vi "Begin.vi"() -> (0 "error out":errorcluster)   [LabVIEW 2012]
doc: "Called before other user functions, this VI is expected to open initial I/O refnums, load in file data, and do all program initialization. Notice that the <B>error out</B> terminal is simply used for data flow. Wiring it to other structures or subVIs ensures that this VI runs first."
uses:
  <vilib>/Rock Robotics/WPI/DriverStation/WPI_DriverStationRobotMode2.ctl
  <vilib>/Rock Robotics/WPI/Joystick/WPI_JoystickDeviceEnum.ctl
  <vilib>/Rock Robotics/WPI/Solenoid/WPI_SolenoidChannel.ctl
  <vilib>/Rock Robotics/SystemInterfaces/DIO/FPGA_DIORelayChannel.ctl
  <vilib>/Rock Robotics/WPI/Relay/WPI_RelayDirection.ctl
  <vilib>/Rock Robotics/SystemInterfaces/DIO/FPGA_DIOChannel.ctl
  <vilib>/Rock Robotics/WPI/Encoder/WPI_EncoderType.ctl
  <vilib>/Rock Robotics/SystemInterfaces/DIO/FPGA_DIOPWMChannel.ctl
  <vilib>/Rock Robotics/SystemInterfaces/AI/FPGA_AIGyroChannel.ctl
  <vilib>/Rock Robotics/SystemInterfaces/Typedef/FPGA_TypedefSolenoidModule.ctl
  Robot Global Data.vi
  <vilib>/Rock Robotics/WPI/Solenoid/WPI_SolenoidOpenSingle.vi
  <vilib>/Rock Robotics/WPI/Solenoid/Deprecated/WPI_SolenoidSetBool.vi
  <vilib>/Rock Robotics/WPI/Counter/WPI_CounterDigitalInputToDigitalSource.vi
  <vilib>/Rock Robotics/WPI/MotorControl/WPI_MotorControlOpen Jaguar.vi
  <vilib>/Rock Robotics/WPI/RobotDrive/WPI_RobotDriveOpen4MotorWithTalon.vi
  <vilib>/Rock Robotics/WPI/Compressor/WPI_CompressorGetSetRefNum.vi
  <vilib>/Rock Robotics/WPI/MotorControl/WPI_MotorControlOpen Talon.vi
  <vilib>/Rock Robotics/WPI/RobotDrive/WPI_RobotDriveOpen4MotorWithExistingMotors.vi
  <vilib>/Rock Robotics/WPI/MotorControl/WPI_MotorControlOpen Victor.vi
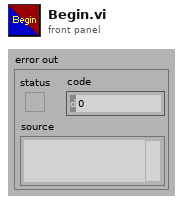
[diagram p1: front panel]
types:
  T1 = typedef "FPGA_DIOChannel.ctl" = enum8{"DIO 1", "DIO 2", "DIO 3", "DIO 4", "DIO 5", "DIO 6", "DIO 7", "DIO 8", "DIO 9", "DIO 10", "DIO 11", "DIO 12", "DIO 13", "DIO 14", "Invalid"}
  T2 = typedef "WPI_SolenoidChannel.ctl" = enum8{"Solenoid 1", "Solenoid 2", "Solenoid 3", "Solenoid 4", "Solenoid 5", "Solenoid 6", "Solenoid 7", "Solenoid 8", "Invalid"}
  T3 = typedef "FPGA_TypedefSolenoidModule.ctl" = enum16{"Solenoid Module 1", "Solenoid Module 2"}
  T4 = typedef "FPGA_AIGyroChannel.ctl" = enum8{"AI 1", "AI 2", "Invalid"}
  T5 = typedef "WPI_EncoderType.ctl" = enum16{"1x", "2x", "4x"}
  T6 = typedef "FPGA_DIORelayChannel.ctl" = enum8{"Relay 1", "Relay 2", "Relay 3", "Relay 4", "Relay 5", "Relay 6", "Relay 7", "Relay 8", "Invalid"}
  T7 = typedef "WPI_JoystickDeviceEnum.ctl" = enum16{"USB 1", "USB 2", "USB 3", "USB 4", "Kinect 1", "Kinect 2"}
  T8 = typedef "FPGA_DIOPWMChannel.ctl" = enum8{"PWM 1", "PWM 2", "PWM 3", "PWM 4", "PWM 5", "PWM 6", "PWM 7", "PWM 8", "PWM 9", "PWM 10", "Invalid"}
  T9 = typedef "WPI_RelayDirection.ctl" = enum16{"Both directions", "Forward only", "Reverse only"}
  T10 = typedef "WPI_DriverStationRobotMode2.ctl" = enum16{"Autonomous Disabled", "Autonomous Enabled", "Teleop Disabled", "Teleop Enabled", "Timeout", "Finish", "Test Disabled", "Test Enabled"}
  T11 = typedef "WPI_RobotDriveDevRef.ctl" = cluster{"DevStatus":errorcluster, "Motors[]":T12[], "Square Inputs":bool, "Max Output":dbl, "Isochronous":bool}
  T12 = typedef "WPI_MotorControlDeviceRef.ctl" = cluster{"DeviceStatus":errorcluster, "Type":enum16{"PWM", "CAN"}, "PWM":cluster{"Digital Module":T13, "PWM Channel":T8, "DeadBand":T14}, "CAN":cluster{"Device Number":u8, "Control Mode":T15, "Semaphore":T16, "Max Vout":dbl}, "Invert":bool, "TransformRef":T17, "InvTransformRef":T17}
  T13 = typedef "FPGA_TypedefDigitalModule.ctl" = enum16{"Digital Module 1", "Digital Module 2"}
  T14 = typedef "WPI_PWMDeadband.ctl" = cluster{"Name":string, "maxPositivePwm":i32, "minPositivePwm":i32, "centerPwm":i32, "maxNegativePwm":i32, "minNegativePwm":i32, "angularRange":u16}
  T15 = typedef "WPI_CANJaguar_ControlMode.ctl" = enum8{"Percent VBus", "Current", "Speed", "Position", "Voltage"}
  T16 = typedef "Semaphore RefNum" = refnum<k1>
  T17 = typedef "WPI_PWMTransform_ConPane.ctl" = refnum<vi>
  T18 = typedef "WPI_DigitalInputDevRef.ctl" = cluster{"DevStatus":errorcluster, "DIO Channel":T1, "Digital Module":T13}
  T19 = typedef "WPI_CompressorDevRef.ctl" = cluster{"DevStatus":errorcluster, "DigitalInputDevRef":T18, "RelayDevRef":T20}
  T20 = typedef "WPI_RelayDevRef.ctl" = cluster{"DevStatus":errorcluster, "Relay Channel":T6, "Digital Module":T13, "Relay Direction":T9}
  T21 = typedef "WPI_JoystickDevRef.ctl" = cluster{"Device":T7}
  T22 = typedef "WPI_SolenoidDevRef.ctl" = cluster{"DevStatus":errorcluster, "Solenoid Module":T3, "Forward Solenoid Channel":T2, "Reverse Solenoid Channel":T2}
  T23 = typedef "FPGA_CounterEncoderSourceConvertionLVSourceType.ctl" = cluster{"DevStatus":errorcluster, "AnalogTriggerMode?":bool, "DigitalMode":cluster{"Digital Module":T13, "DIO Channel":T24}, "AnalogTriggerMode":cluster{"AnalogTriggerIndex":T25, "OutputType":T26}}
  T24 = typedef "FPGA_DIODigitalSourceChannel.ctl" = enum8{"DIO 1", "DIO 2", "DIO 3", "DIO 4", "DIO 5", "DIO 6", "DIO 7", "DIO 8", "DIO 9", "DIO 10", "DIO 11", "DIO 12", "DIO 13", "DIO 14", "Disabled"}
  T25 = typedef "FPGA_AnalogTriggerIndex.ctl" = enum8{"Trig 0", "Trig 1", "Trig 2", "Trig 3", "Trig 4", "Trig 5", "Trig 6", "Trig 7", "Invalid"}
  T26 = typedef "FPGA_AnalogTriggerOutType.ctl" = enum16{"InWindow", "TriggerState", "Rising", "Falling"}
  T27 = typedef "WPI_GyroDevRef.ctl" = cluster{"DevStatus":errorcluster, "Analog Module":T28, "Analog Channel":T29, "Offset":dbl, "Gain (VoltsPerDegree/Second)":dbl}
  T28 = typedef "FPGA_TypedefAnalogModule.ctl" = enum16{"Analog Module 1", "Analog Module 2"}
  T29 = typedef "FPGA_AIChannel.ctl" = enum8{"AI 1", "AI 2", "AI 3", "AI 4", "AI 5", "AI 6", "AI 7", "AI 8", "Invalid"}
  T30 = typedef "WPI_EncoderDevRef.ctl" = cluster{"DevStatus":errorcluster, "EncoderIndex":T31, "CounterIndex":T32, "DistancePerCount":dbl, "Decoding Type":T5}
  T31 = typedef "FPGA_EncoderIdx.ctl" = enum8{"Enc 0", "Enc 1", "Enc 2", "Enc 3", "Invalid"}
  T32 = typedef "FPGA_CounterCtrSystemIndex.ctl" = enum8{"Ctr 0", "Ctr 1", "Ctr 2", "Ctr 3", "Ctr 4", "Ctr 5", "Ctr 6", "Ctr 7", "Invalid"}
  T33 = cluster{"Target Voltage":dbl, "Target Speed":dbl, "Angle Up?":bool}
  T34 = cluster{"Target Voltage":dbl, "Target Speed":i32, "Angle Up?":bool}
  T35 = cluster{"Target Voltage":i32, "Target Speed":i32, "Angle Up?":bool}
  T36 = cluster{"Target Voltage":dbl, "Target Speed":dbl, "Angle Up?":bool}[]
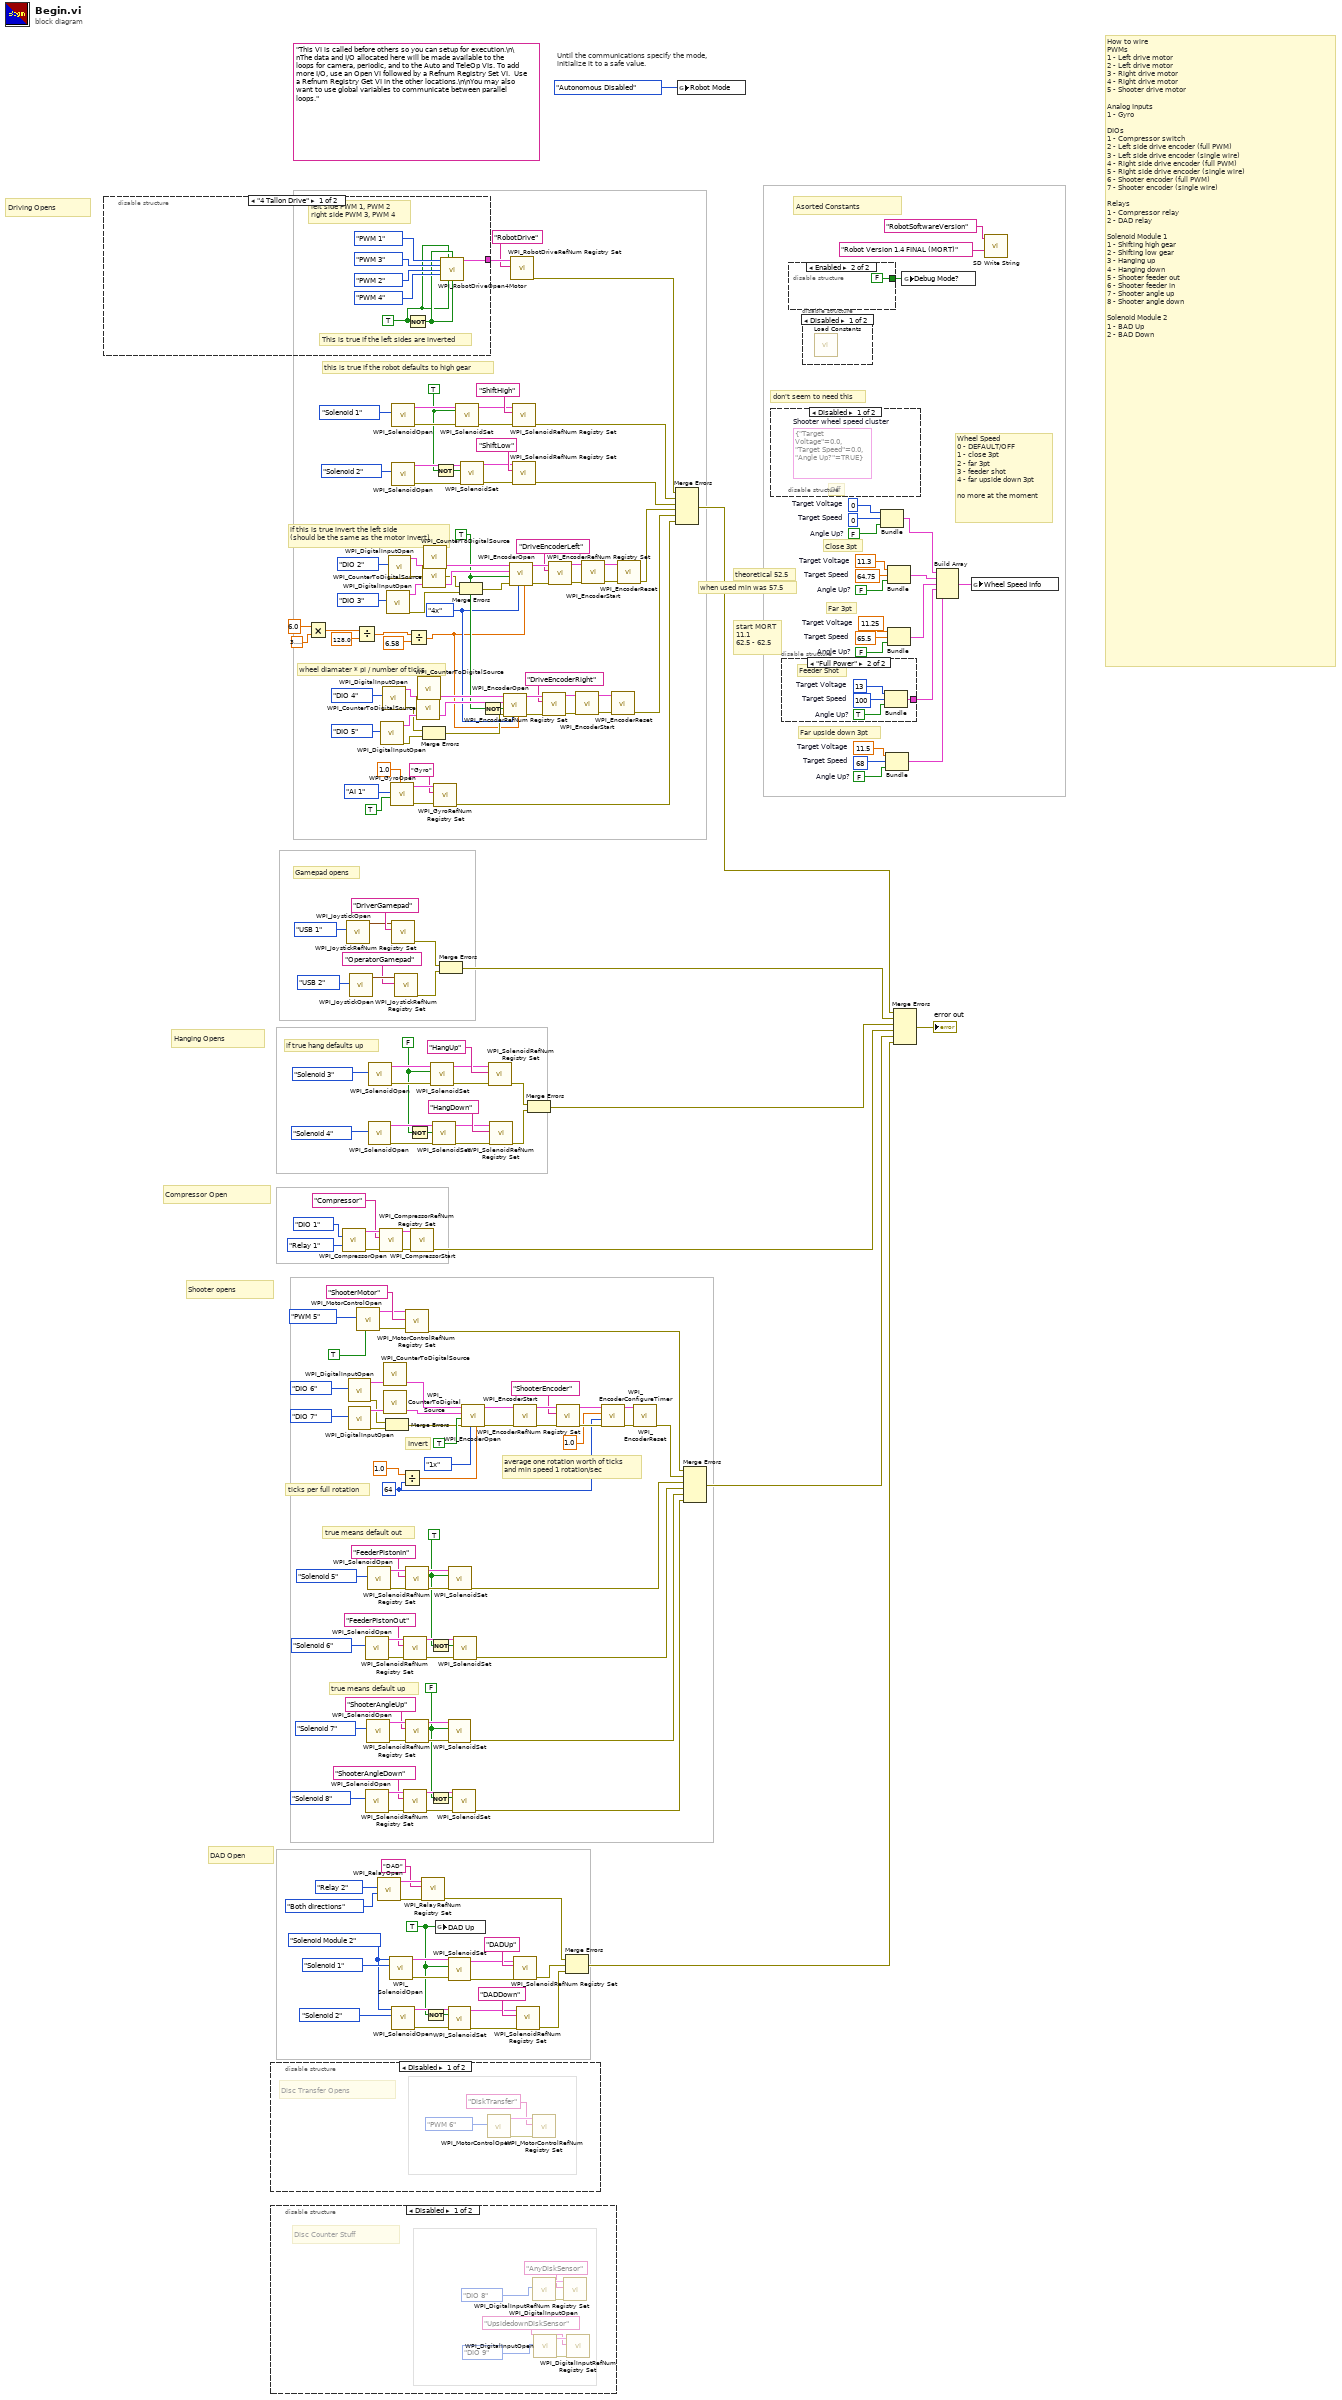
[diagram p0: block diagram]
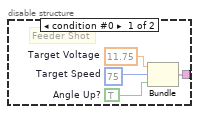
[diagram p3: hidden frame]
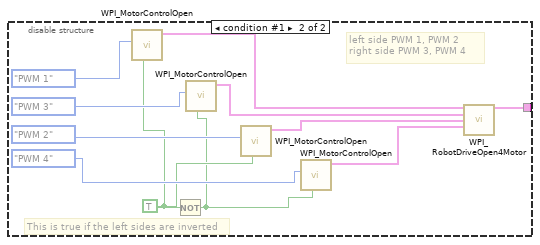
[diagram p4: hidden frame]
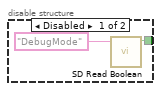
[diagram p5: hidden frame]
diagram:
  w6 = FALSE  # Angle Up?
  w5 = 65.5  # Target Speed
  w4 = 11.25  # Target Voltage
  w10 = FALSE  # Angle Up?
  w9 = 68  # Target Speed
  w8 = 11.5  # Target Voltage
  w14 = FALSE  # Angle Up?
  w13 = 0  # Target Speed
  w12 = 0  # Target Voltage
  w16 = u8 64 ("Number Samples to Average")
  w23 = FALSE  # Angle Up?
  w24 = 64.75  # Target Speed
  w25 = 11.3  # Target Voltage
  w84 = FALSE
  w98 = TRUE
  w60 = TRUE
  w62 = FPGA_TypedefSolenoidModule."Solenoid Module 2" ("Solenoid Module (Module 1)")
  w63 = FALSE
  w65 = WPI_EncoderType."4x" ("Decoding Type")
  w66 = TRUE ("Invert Direction (False)")
  w82 = TRUE
  (unwired) "This VI is called before others so you can setup for execution.\n\nThe data and I/O allocated here will be made available to the loops for camera, periodic, and to the Auto and TeleOp VIs. To add more I/O, use an Open VI followed by a Refnum Registry Set VI.  Use a Refnum Registry Get VI in the other locations.\n\nYou may also want to use global variables to communicate between parallel loops."
  # "start MORT\n11.1\n62.5 - 62.5"
  # "when used min was 57.5"
  # "theoretical 52.5"
  # "don't seem to need this"
  # "Far 3pt"
  # "Far upside down 3pt"
  # "average one rotation worth of ticks\nand min speed 1 rotation/sec"
  # "Close 3pt"
  # "How to wire\nPWMs\n1 - Left drive motor\n2 - Left drive motor\n3 - Right drive motor\n4 - Right drive motor\n5 - Shooter drive motor\n\nAnalog Inputs\n1 - Gyro\n\nDIOs\n1 - Compressor switch\n2 - Left side drive encoder (full PWM)\n3 - Left side drive encoder (single wire)\n4 - Right side drive encoder (full PWM)\n5 - Right side drive encoder (single wire)\n6 - Shooter encoder (full PWM)\n7 - Shooter encoder (single wire)\n\nRelays\n1 - Compressor relay\n2 - DAD relay\n\nSolenoid Module 1\n1 - Shifting high gear\n2 - Shifting low gear\n3 - Hanging up\n4 - Hanging down\n5 - Shooter feeder out\n6 - Shooter feeder in\n7 - Shooter angle up\n8 - Shooter angle down\n\nSolenoid Module 2\n1 - BAD Up\n2 - BAD Down"
  # "Asorted Constants"
  # "true means default up"
  # "true means default out"
  # "if true hang defaults up"
  # "Gamepad opens"
  # "wheel diamater * pi / number of ticks"
  # "if this is true invert the left side\n(should be the same as the motor invert)"
  # "this is true if the robot defaults to high gear"
  # "Compressor Open"
  # "Wheel Speed\n0 - DEFAULT/OFF\n1 - close 3pt\n2 - far 3pt\n3 - feeder shot\n4 - far upside down 3pt\n\nno more at the moment"
  # "DAD Open"
  # "Hanging Opens"
  # "Driving Opens"
  # "Shooter opens"
  # "Invert"
  # "ticks per full rotation"
  # "Until the communications specify the mode,\ninitialize it to a safe value."
  n1 = disable-structure shown="\"4 Tallon Drive\"" {
    disable-tunnel: [w219 w234] -> w212
    frame condition #0 (active) {
      w217 = TRUE ("Rear Left Motor Inverted")
      # "left side PWM 1, PWM 2\nright side PWM 3, PWM 4"
      # "This is true if the left sides are inverted"
      n2 = Not(x=w217) -> (.not. x?=w218:bool)
      n3 = call-poly <vilib>:"WPI_RobotDriveOpen4Motor.vi"("Rear Left Motor"=FPGA_DIOPWMChannel."PWM 1", "Rear Left Motor Inverted"=w217, "Rear Right Motor Inverted"=w218, "Rear Right Motor"=FPGA_DIOPWMChannel."PWM 3", "Front Left Motor"=FPGA_DIOPWMChannel."PWM 2", "Front Right Motor"=FPGA_DIOPWMChannel."PWM 4" ("Front Left Motor"), "Front Left Motor Inverted"=w217, "Front Right Motor Inverted"=w218) -> ("RobotDriveDevRef"=w219:T11)  [unwired: 6 in, 1 out]
    }
    frame condition #1 {
      w229 = TRUE ("Rear Left Motor Inverted")
      # "left side PWM 1, PWM 2\nright side PWM 3, PWM 4"
      # "This is true if the left sides are inverted"
      n4 = call-poly <vilib>:"WPI_MotorControlOpen.vi"("Invert"=w229, "PWM Channel"=FPGA_DIOPWMChannel."PWM 1" ("Rear Left Motor")) -> ("MotorControlDeviceRef"=w227:T12)  [unwired: 8 in, 1 out]
      n5 = Not(x=w229) -> (.not. x?=w228:bool)
      n6 = call-poly <vilib>:"WPI_MotorControlOpen.vi"("Invert"=w228, "PWM Channel"=FPGA_DIOPWMChannel."PWM 3" ("Rear Right Motor")) -> ("MotorControlDeviceRef"=w226:T12)  [unwired: 8 in, 1 out]
      n7 = call-poly <vilib>:"WPI_MotorControlOpen.vi"("Invert"=w229, "PWM Channel"=FPGA_DIOPWMChannel."PWM 2" ("Front Left Motor")) -> ("MotorControlDeviceRef"=w225:T12)  [unwired: 8 in, 1 out]
      n8 = call-poly <vilib>:"WPI_MotorControlOpen.vi"("Invert"=w228, "PWM Channel"=FPGA_DIOPWMChannel."PWM 4" ("Front Left Motor")) -> ("MotorControlDeviceRef"=w224:T12)  [unwired: 8 in, 1 out]
      n9 = call-poly <vilib>:"WPI_RobotDriveOpen4Motor.vi"("Rear Left Motor Dev Ref"=w227, "Rear Right Motor Dev Ref"=w226, "Front Left Motor Dev Ref"=w225, "Front Right Motor Dev Ref"=w224) -> ("RobotDriveDevRef"=w234:T11)  [unwired: 10 in, 1 out]
    }
  }
  n10 = disable-structure shown="Disabled" {
    frame Disabled {
      # "Disc Transfer Opens"
      n11 = call-poly <vilib>:"WPI_MotorControlOpen.vi"("PWM Channel"=FPGA_DIOPWMChannel."PWM 6") -> ("error out"=w236:errorcluster, "MotorControlDeviceRef"=w237:T12)  [unwired: 9 in]
      n12 = call <vilib>:"WPI_MotorControlRefNum Registry Set.vi"("error in (no error)"=w236, "refnum name"="DiskTransfer", "MotorControlDevRef"=w237) -> ()  [unwired: 7 in, 2 out]
    }
    frame Enabled {
    }
  }
  n13 = disable-structure shown="Disabled" {
    frame Disabled {
      # "Disc Counter Stuff"
      n14 = call <vilib>:"WPI_DigitalInputOpen.vi"("DIO Channel"=FPGA_DIOChannel."DIO 8") -> ("error out"=w246:errorcluster, "DigitalInputDevRef"=w245:T18)  [unwired: 9 in]
      n15 = call <vilib>:"WPI_DigitalInputOpen.vi"("DIO Channel"=FPGA_DIOChannel."DIO 9") -> ("error out"=w244:errorcluster, "DigitalInputDevRef"=w243:T18)  [unwired: 9 in]
      n16 = call <vilib>:"WPI_DigitalInputRefNum Registry Set.vi"("error in (no error)"=w246, "refnum name"="AnyDiskSensor", "DigitalInputDevRef"=w245) -> ()  [unwired: 7 in, 2 out]
      n17 = call <vilib>:"WPI_DigitalInputRefNum Registry Set.vi"("error in (no error)"=w244, "refnum name"="UpsidedownDiskSensor", "DigitalInputDevRef"=w243) -> ()  [unwired: 7 in, 2 out]
    }
    frame Enabled {
    }
  }
  n18 = Multiply(x=6.0, y=3.141592653589793) -> (x*y=w151:dbl)
  n19 = call <vilib>:"WPI_CompressorOpen.vi"("Pressure Switch DIO Channel"=FPGA_DIOChannel."DIO 1", "Relay Channel"=FPGA_DIORelayChannel."Relay 1") -> ("CompressorDevRef"=w164:T19, "error out"=w162:errorcluster)  [unwired: 12 in]
  n20 = call <vilib>:"WPI_JoystickOpen.vi"("JoystickDevice"=WPI_JoystickDeviceEnum."USB 1") -> ("JoystickDevRef"=w214:T21)  [unwired: 10 in]
  n21 = call <vilib>:"WPI_DigitalInputOpen.vi"("DIO Channel"=FPGA_DIOChannel."DIO 6") -> ("error out"=w180:errorcluster, "DigitalInputDevRef"=w193:T18)  [unwired: 9 in]
  n22 = call <vilib>:"WPI_DigitalInputOpen.vi"("DIO Channel"=FPGA_DIOChannel."DIO 7") -> ("error out"=w179:errorcluster, "DigitalInputDevRef"=w189:T18)  [unwired: 9 in]
  n23 = call <vilib>:"WPI_JoystickOpen.vi"("JoystickDevice"=WPI_JoystickDeviceEnum."USB 2") -> ("JoystickDevRef"=w166:T21)  [unwired: 10 in]
  n24 = Divide(x=w151, y=128.0 ("x")) -> (x/y=w2:dbl)
  n25 = call-poly <vilib>:"WPI_MotorControlOpen.vi"("Invert"=TRUE, "PWM Channel"=FPGA_DIOPWMChannel."PWM 5") -> ("error out"=w173:errorcluster, "MotorControlDeviceRef"=w174:T12)  [unwired: 8 in]
  n26 = call-poly <vilib>:"WPI_SolenoidOpen.vi"("Solenoid Channel"=WPI_SolenoidChannel."Solenoid 8") -> ("error out"=w94:errorcluster, "SolenoidDevRef"=w93:T22)  [unwired: 9 in]
  n27 = call-poly <vilib>:"WPI_SolenoidOpen.vi"("Solenoid Channel"=WPI_SolenoidChannel."Solenoid 6") -> ("error out"=w108:errorcluster, "SolenoidDevRef"=w107:T22)  [unwired: 9 in]
  n28 = call-poly <vilib>:"WPI_SolenoidOpen.vi"("Solenoid Channel"=WPI_SolenoidChannel."Solenoid 7") -> ("error out"=w89:errorcluster, "SolenoidDevRef"=w90:T22)  [unwired: 9 in]
  n29 = call-poly <vilib>:"WPI_SolenoidOpen.vi"("Solenoid Channel"=WPI_SolenoidChannel."Solenoid 5") -> ("error out"=w103:errorcluster, "SolenoidDevRef"=w104:T22)  [unwired: 9 in]
  n30 = call-poly <vilib>:"WPI_SolenoidOpen.vi"("Solenoid Channel"=WPI_SolenoidChannel."Solenoid 4") -> ("error out"=w130:errorcluster, "SolenoidDevRef"=w131:T22)  [unwired: 9 in]
  n31 = call-poly <vilib>:"WPI_SolenoidOpen.vi"("Solenoid Channel"=WPI_SolenoidChannel."Solenoid 3") -> ("error out"=w133:errorcluster, "SolenoidDevRef"=w132:T22)  [unwired: 9 in]
  n32 = call <vilib>:"WPI_RelayOpen.vi"("Relay Direction"=WPI_RelayDirection."Both directions", "Relay Channel"=FPGA_DIORelayChannel."Relay 2") -> ("error out"=w196:errorcluster, "RelayDevRef"=w195:T20)  [unwired: 8 in]
  n33 = call <vilib>:"WPI_CompressorRefNum Registry Set.vi"("error in (no error)"=w162, "refnum name"="Compressor", "CompressorDevRef"=w164) -> ("error out"=w112:errorcluster, "CompressorDevRef"=w113:T19)  [unwired: 7 in]
  n34 = call <vilib>:"WPI_DigitalInputOpen.vi"("DIO Channel"=FPGA_DIOChannel."DIO 5") -> ("error out"=w53:errorcluster, "DigitalInputDevRef"=w74:T18)  [unwired: 9 in]
  n35 = call <vilib>:"WPI_DigitalInputOpen.vi"("DIO Channel"=FPGA_DIOChannel."DIO 4") -> ("error out"=w52:errorcluster, "DigitalInputDevRef"=w73:T18)  [unwired: 9 in]
  n36 = call-poly <vilib>:"WPI_CounterToDigitalSource.vi"("DigitalInputDevRef"=w193) -> ("Digital Source"=w192:T23)  [unwired: 6 in]
  n37 = call-poly <vilib>:"WPI_CounterToDigitalSource.vi"("DigitalInputDevRef"=w189) -> ("Digital Source"=w186:T23)  [unwired: 6 in]
  n38 = Merge Errors(w180, w179) -> (w181:errorcluster)
  n39 = call <vilib>:"WPI_DigitalInputOpen.vi"("DIO Channel"=FPGA_DIOChannel."DIO 3") -> ("error out"=w48:errorcluster, "DigitalInputDevRef"=w154:T18)  [unwired: 9 in]
  n40 = call <vilib>:"WPI_DigitalInputOpen.vi"("DIO Channel"=FPGA_DIOChannel."DIO 2") -> ("error out"=w49:errorcluster, "DigitalInputDevRef"=w155:T18)  [unwired: 9 in]
  n41 = call-poly <vilib>:"WPI_SolenoidOpen.vi"("Solenoid Channel"=WPI_SolenoidChannel."Solenoid 1", "Solenoid Module (Module 1)"=w62) -> ("error out"=w117:errorcluster, "SolenoidDevRef"=w121:T22)  [unwired: 8 in]
  n42 = call <vilib>:"WPI_GyroOpen.vi"("Calibration Time (s)"=1.0, "Calibrate On Open"=TRUE, "Analog Channel"=FPGA_AIGyroChannel."AI 1") -> ("error out"=w143:errorcluster, "GyroDevRef"=w142:T27)  [unwired: 6 in, 1 out]
  n43 = call-poly <vilib>:"WPI_SolenoidOpen.vi"("Solenoid Channel"=WPI_SolenoidChannel."Solenoid 1") -> ("error out"=w203:errorcluster, "SolenoidDevRef"=w206:T22)  [unwired: 9 in]
  n44 = call-poly <vilib>:"WPI_SolenoidOpen.vi"("Solenoid Channel"=WPI_SolenoidChannel."Solenoid 2") -> ("error out"=w200:errorcluster, "SolenoidDevRef"=w202:T22)  [unwired: 9 in]
  n45 = call <vilib>:"WPI_JoystickRefNum Registry Set.vi"("refnum name"="DriverGamepad", "JoystickDevRef"=w214) -> ("error out"=w45:errorcluster)  [unwired: 8 in, 1 out]
  n46 = call-poly <vilib>:"WPI_SolenoidOpen.vi"("Solenoid Channel"=WPI_SolenoidChannel."Solenoid 2", "Solenoid Module (Module 1)"=w62) -> ("error out"=w114:errorcluster, "SolenoidDevRef"=w119:T22)  [unwired: 8 in]
  n47 = call <vilib>:"WPI_JoystickRefNum Registry Set.vi"("refnum name"="OperatorGamepad", "JoystickDevRef"=w166) -> ("error out"=w44:errorcluster)  [unwired: 8 in, 1 out]
  n48 = Divide(x=1.0, y=w16) -> (x/y=w17:dbl)
  n49 = call <vilib>:"WPI_SolenoidRefNum Registry Set.vi"("error in (no error)"=w108, "refnum name"="FeederPistonOut", "SolenoidDevRef"=w107) -> ("error out"=w110:errorcluster, "SolenoidDevRef"=w109:T22)  [unwired: 7 in]
  n50 = call <vilib>:"WPI_SolenoidRefNum Registry Set.vi"("error in (no error)"=w94, "refnum name"="ShooterAngleDown", "SolenoidDevRef"=w93) -> ("error out"=w96:errorcluster, "SolenoidDevRef"=w95:T22)  [unwired: 7 in]
  n51 = call <vilib>:"WPI_MotorControlRefNum Registry Set.vi"("error in (no error)"=w173, "refnum name"="ShooterMotor", "MotorControlDevRef"=w174) -> ("error out"=w41:errorcluster)  [unwired: 7 in, 1 out]
  n52 = call <vilib>:"WPI_SolenoidRefNum Registry Set.vi"("error in (no error)"=w103, "refnum name"="FeederPistonIn", "SolenoidDevRef"=w104) -> ("error out"=w101:errorcluster, "SolenoidDevRef"=w102:T22)  [unwired: 7 in]
  n53 = call <vilib>:"WPI_SolenoidRefNum Registry Set.vi"("error in (no error)"=w89, "refnum name"="ShooterAngleUp", "SolenoidDevRef"=w90) -> ("error out"=w87:errorcluster, "SolenoidDevRef"=w88:T22)  [unwired: 7 in]
  n54 = Divide(x=w2, y=6.58 ("x")) -> (x/y=w3:dbl)
  n55 = Not(x=w63) -> (.not. x?=w64:bool)
  n56 = call <vilib>:"WPI_CompressorStart.vi"("error in (no error)"=w112, "CompressorDevRef"=w113) -> ("error out"=w29:errorcluster)  [unwired: 8 in, 1 out]
  n57 = call-poly <vilib>:"WPI_CounterToDigitalSource.vi"("DigitalInputDevRef"=w74) -> ("Digital Source"=w71:T23)  [unwired: 6 in]
  n58 = call-poly <vilib>:"WPI_CounterToDigitalSource.vi"("DigitalInputDevRef"=w73) -> ("Digital Source"=w69:T23)  [unwired: 6 in]
  n59 = call <vilib>:"WPI_RelayRefNum Registry Set.vi"("error in (no error)"=w196, "refnum name"="DAD", "RelayDevRef"=w195) -> ("error out"=w35:errorcluster)  [unwired: 7 in, 1 out]
  n60 = Merge Errors(w52, w53) -> (w51:errorcluster)
  n61 = call-poly <vilib>:"WPI_CounterToDigitalSource.vi"("DigitalInputDevRef"=w154) -> ("Digital Source"=w157:T23)  [unwired: 6 in]
  n62 = call-poly <vilib>:"WPI_CounterToDigitalSource.vi"("DigitalInputDevRef"=w155) -> ("Digital Source"=w159:T23)  [unwired: 6 in]
  n63 = Not(x=w60) -> (.not. x?=w61:bool)
  n64 = Not(x=w84) -> (.not. x?=w97:bool)
  n65 = Not(x=w98) -> (.not. x?=w111:bool)
  n66 = call-poly <vilib>:"WPI_SolenoidSet.vi"("error in (no error)"=w133, "Value"=w63, "SolenoidDevRef"=w132) -> ("error out"=w126:errorcluster, "SolenoidDevRef"=w129:T22)  [unwired: 7 in]
  n67 = call-poly <vilib>:"WPI_SolenoidSet.vi"("error in (no error)"=w130, "Value"=w64, "SolenoidDevRef"=w131) -> ("error out"=w127:errorcluster, "SolenoidDevRef"=w128:T22)  [unwired: 7 in]
  n68 = Not(x=w82) -> (.not. x?=w83:bool)
  n69 = call <vilib>:"WPI_GyroRefNum Registry Set.vi"("error in (no error)"=w143, "refnum name"="Gyro", "GyroDevRef"=w142) -> ("error out"=w46:errorcluster)  [unwired: 7 in, 1 out]
  n70 = global write "Robot Global Data.vi" "DAD Up"(w60) -> ()
  n71 = Merge Errors(w45, w44) -> (w31:errorcluster)
  n72 = call-poly <vilib>:"WPI_SolenoidSet.vi"("error in (no error)"=w87, "Value"=w84, "SolenoidDevRef"=w88) -> ("error out"=w37:errorcluster)  [unwired: 7 in, 1 out]
  n73 = call-poly <vilib>:"WPI_SolenoidSet.vi"("error in (no error)"=w117, "Value"=w60, "SolenoidDevRef"=w121) -> ("error out"=w116:errorcluster, "SolenoidDevRef"=w120:T22)  [unwired: 7 in]
  n74 = call-poly <vilib>:"WPI_SolenoidSet.vi"("error in (no error)"=w114, "Value"=w61, "SolenoidDevRef"=w119) -> ("error out"=w115:errorcluster, "SolenoidDevRef"=w118:T22)  [unwired: 7 in]
  n75 = call-poly <vilib>:"WPI_SolenoidSet.vi"("error in (no error)"=w101, "Value"=w98, "SolenoidDevRef"=w102) -> ("error out"=w39:errorcluster)  [unwired: 7 in, 1 out]
  n76 = call-poly <vilib>:"WPI_SolenoidSet.vi"("error in (no error)"=w96, "Value"=w97, "SolenoidDevRef"=w95) -> ("error out"=w36:errorcluster)  [unwired: 7 in, 1 out]
  n77 = call-poly <vilib>:"WPI_SolenoidSet.vi"("error in (no error)"=w110, "Value"=w111, "SolenoidDevRef"=w109) -> ("error out"=w38:errorcluster)  [unwired: 7 in, 1 out]
  n78 = call-poly <vilib>:"WPI_SolenoidSet.vi"("error in (no error)"=w203, "Value"=w82, "SolenoidDevRef"=w206) -> ("error out"=w204:errorcluster, "SolenoidDevRef"=w205:T22)  [unwired: 7 in]
  n79 = Merge Errors(w49, w48) -> (w50:errorcluster)
  n80 = call-poly <vilib>:"WPI_SolenoidSet.vi"("error in (no error)"=w200, "Value"=w83, "SolenoidDevRef"=w202) -> ("error out"=w199:errorcluster, "SolenoidDevRef"=w201:T22)  [unwired: 7 in]
  n81 = call <vilib>:"WPI_EncoderOpen.vi"("DistancePerCount"=w17, "Decoding Type"=WPI_EncoderType."1x", "error in (no error)"=w181, "Invert Direction (False)"=TRUE, "BSource"=w186, "ASource"=w192) -> ("error out"=w182:errorcluster, "EncoderDevRef"=w183:T30)  [unwired: 4 in]
  n82 = Not(x=w66) -> (.not. x?=w67:bool)
  n83 = call <vilib>:"WPI_SolenoidRefNum Registry Set.vi"("error in (no error)"=w126, "refnum name"="HangUp", "SolenoidDevRef"=w129) -> ("error out"=w43:errorcluster)  [unwired: 7 in, 1 out]
  n84 = call <vilib>:"WPI_SolenoidRefNum Registry Set.vi"("error in (no error)"=w127, "refnum name"="HangDown", "SolenoidDevRef"=w128) -> ("error out"=w42:errorcluster)  [unwired: 7 in, 1 out]
  n85 = call <vilib>:"WPI_EncoderOpen.vi"("DistancePerCount"=w3, "Decoding Type"=w65, "error in (no error)"=w51, "Invert Direction (False)"=w67, "BSource"=w71, "ASource"=w69) -> ("error out"=w75:errorcluster, "EncoderDevRef"=w76:T30)  [unwired: 4 in]
  n86 = call <vilib>:"WPI_EncoderOpen.vi"("DistancePerCount"=w3, "Decoding Type"=w65, "error in (no error)"=w50, "Invert Direction (False)"=w66, "BSource"=w157, "ASource"=w159) -> ("error out"=w150:errorcluster, "EncoderDevRef"=w149:T30)  [unwired: 4 in]
  n87 = call <vilib>:"WPI_RobotDriveRefNum Registry Set.vi"("refnum name"="RobotDrive", "RobotDriveDevRef"=w212) -> ("error out"=w57:errorcluster)  [unwired: 8 in, 1 out]
  n88 = call <vilib>:"WPI_SolenoidRefNum Registry Set.vi"("error in (no error)"=w204, "refnum name"="ShiftHigh", "SolenoidDevRef"=w205) -> ("error out"=w56:errorcluster)  [unwired: 7 in, 1 out]
  n89 = call <vilib>:"WPI_SolenoidRefNum Registry Set.vi"("error in (no error)"=w199, "refnum name"="ShiftLow", "SolenoidDevRef"=w201) -> ("error out"=w55:errorcluster)  [unwired: 7 in, 1 out]
  n90 = call <vilib>:"WPI_EncoderStart.vi"("error in (no error)"=w182, "EncoderDevRef"=w183) -> ("error out"=w178:errorcluster, "EncoderDevRef"=w184:T30)  [unwired: 8 in]
  n91 = call <vilib>:"WPI_SolenoidRefNum Registry Set.vi"("error in (no error)"=w116, "refnum name"="DADUp", "SolenoidDevRef"=w120) -> ("error out"=w34:errorcluster)  [unwired: 7 in, 1 out]
  n92 = call <vilib>:"WPI_SolenoidRefNum Registry Set.vi"("error in (no error)"=w115, "refnum name"="DADDown", "SolenoidDevRef"=w118) -> ("error out"=w33:errorcluster)  [unwired: 7 in, 1 out]
  n93 = Merge Errors(w43, w42) -> (w30:errorcluster)
  n94 = call <vilib>:"WPI_EncoderRefNum Registry Set.vi"("error in (no error)"=w75, "refnum name"="DriveEncoderRight", "EncoderDevRef"=w76) -> ("error out"=w77:errorcluster, "EncoderDevRef"=w78:T30)  [unwired: 7 in]
  n95 = call <vilib>:"WPI_EncoderRefNum Registry Set.vi"("error in (no error)"=w150, "refnum name"="DriveEncoderLeft", "EncoderDevRef"=w149) -> ("error out"=w148:errorcluster, "EncoderDevRef"=w147:T30)  [unwired: 7 in]
  n96 = call <vilib>:"WPI_EncoderRefNum Registry Set.vi"("error in (no error)"=w178, "refnum name"="ShooterEncoder", "EncoderDevRef"=w184) -> ("error out"=w169:errorcluster, "EncoderDevRef"=w170:T30)  [unwired: 7 in]
  n97 = Merge Errors(w35, w34, w33) -> (w27:errorcluster)
  n98 = call <vilib>:"WPI_EncoderStart.vi"("error in (no error)"=w77, "EncoderDevRef"=w78) -> ("error out"=w79:errorcluster, "EncoderDevRef"=w80:T30)  [unwired: 8 in]
  n99 = call <vilib>:"WPI_EncoderStart.vi"("error in (no error)"=w148, "EncoderDevRef"=w147) -> ("error out"=w146:errorcluster, "EncoderDevRef"=w145:T30)  [unwired: 8 in]
  n100 = call <vilib>:"WPI_EncoderConfigureTimer.vi"("error in (no error)"=w169, "Number Samples to Average"=w16, "Minimum Rate"=1.0, "EncoderDevRef"=w170) -> ("error out"=w172:errorcluster, "EncoderDevRef"=w171:T30)  [unwired: 6 in]
  n101 = call <vilib>:"WPI_EncoderReset.vi"("error in (no error)"=w79, "EncoderDevRef"=w80) -> ("error out"=w47:errorcluster)  [unwired: 8 in, 1 out]
  n102 = call <vilib>:"WPI_EncoderReset.vi"("error in (no error)"=w146, "EncoderDevRef"=w145) -> ("error out"=w54:errorcluster)  [unwired: 8 in, 1 out]
  n103 = call <vilib>:"WPI_EncoderReset.vi"("error in (no error)"=w172, "EncoderDevRef"=w171) -> ("error out"=w40:errorcluster)  [unwired: 8 in, 1 out]
  n104 = Merge Errors(w57, w56, w55, w54, w47, w46) -> (w32:errorcluster)
  n105 = global write "Robot Global Data.vi" "Robot Mode"(WPI_DriverStationRobotMode2."Autonomous Disabled" ("Robot Mode")) -> ()
  n106 = Merge Errors(w41, w40, w39, w38, w37, w36) -> (w28:errorcluster)
  n107 = disable-structure shown="Disabled" {
    frame Disabled {
      (unwired) T33 {"Target Voltage"=0.0, "Target Speed"=0.0, "Angle Up?"=TRUE}  # Shooter wheel speed cluster
      # "Off"
    }
    frame Enabled {
    }
  }
  n108 = disable-structure shown="\"Full Power\"" {
    disable-tunnel: [w247 w251] -> w20
    frame condition #0 {
      w248 = TRUE  # Angle Up?
      w249 = 75  # Target Speed
      w250 = 11.75  # Target Voltage
      # "Feeder Shot"
      n109 = Bundle("Target Voltage"=w250, "Target Speed"=w249, "Angle Up?"=w248) -> (w247:T34)  [unwired: 1 in]
    }
    frame condition #1 (active) {
      w252 = TRUE  # Angle Up?
      w253 = 100  # Target Speed
      w254 = 13  # Target Voltage
      # "Feeder Shot"
      n110 = Bundle("Target Voltage"=w254, "Target Speed"=w253, "Angle Up?"=w252) -> (w251:T35)  [unwired: 1 in]
    }
  }
  n111 = disable-structure shown="Enabled" {
    disable-tunnel: [w255 FALSE ("Debug Mode?")] -> w18
    frame Disabled {
      n112 = call <vilib>:"SD Read Boolean.vi"("Name"="DebugMode") -> ("Boolean"=w255:bool)  [unwired: 8 in, 2 out]
    }
    frame Enabled {
    }
  }
  n113 = disable-structure shown="Disabled" {
    frame Disabled {
      n114 = call "Load Constants.vi"() -> ()  [unwired: 12 in]
    }
    frame Enabled {
    }
  }
  n115 = Bundle("Target Voltage"=w12, "Target Speed"=w13, "Angle Up?"=w14) -> (w11:T35)  [unwired: 1 in]
  n116 = Bundle("Target Voltage"=w8, "Target Speed"=w9, "Angle Up?"=w10) -> (w7:T34)  [unwired: 1 in]
  n117 = Bundle("Target Voltage"=w25, "Target Speed"=w24, "Angle Up?"=w23) -> (w22:T33)  [unwired: 1 in]
  n118 = Bundle("Target Voltage"=w4, "Target Speed"=w5, "Angle Up?"=w6) -> (w21:T33)  [unwired: 1 in]
  n119 = Merge Errors(w32, w31, w30, w29, w28, w27) -> (→"error out":errorcluster)
  n120 = global write "Robot Global Data.vi" "Debug Mode?"(w18) -> ()
  n121 = Build Array(w11, w22, w21, w20, w7) -> (w19:T36)
  n122 = global write "Robot Global Data.vi" "Wheel Speed Info"(w19) -> ()
  n123 = call <vilib>:"SD Write String.vi"("String"="Robot Version 1.4 FINAL (MORT)", "Name"="RobotSoftwareVersion") -> ()  [unwired: 8 in, 2 out]
